vi "Test Deserialize Floating Point.vi"(8 "error in (no error)":errorcluster) -> (0 "error out":errorcluster)   [LabVIEW 2013]
uses:
  src/Deserializer/JSON Deserializer/JSON Deserializer.lvclass
  <vilib>/addons/_JKI Toolkits/Caraya/classes/Test/Test.lvclass
  <vilib>/addons/_JKI Toolkits/Caraya/classes/Assert/Assert.lvclass
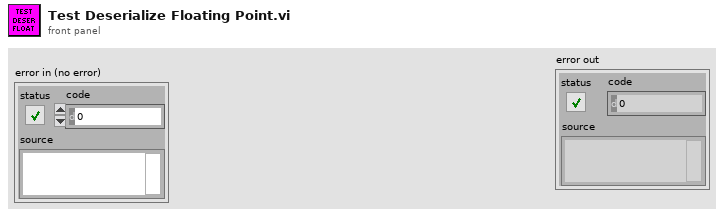
[diagram p1: front panel]
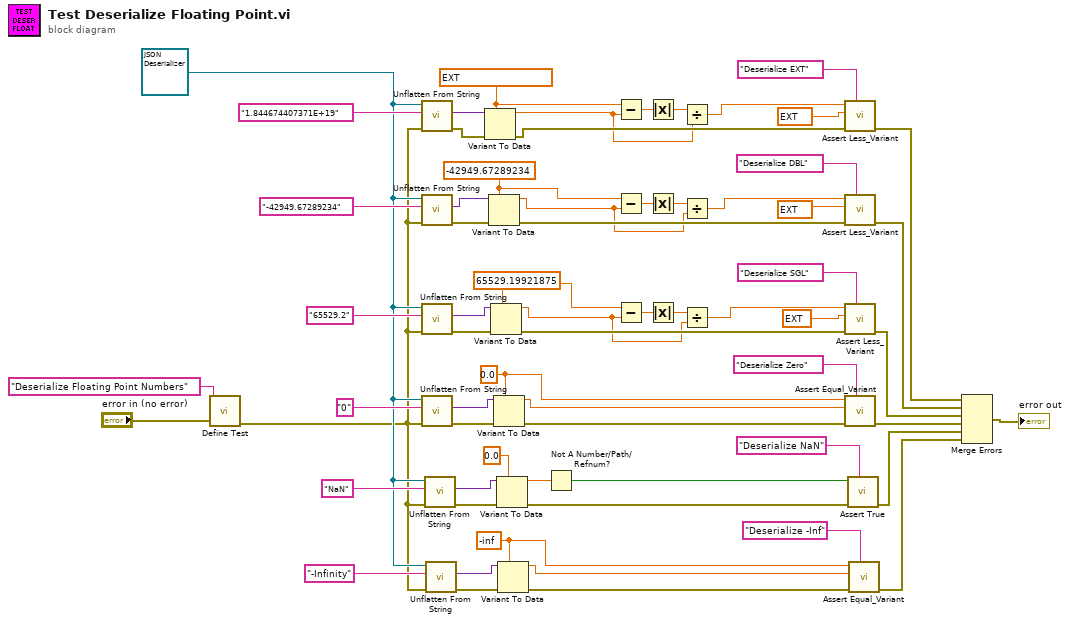
[diagram p0: block diagram]
diagram:
  w8 = -inf ("default (0 DBL)")
  w6 = refnum<class "JSON Deserializer.lvclass"> refnum ("JKI JSON Serialization.lvlib:JSON Deserializer.lvclass")
  w35 = ext 1.844674407371e+19 ("default (0 DBL)")
  w31 = -42949.67289234 ("default (0 DBL)")
  w25 = sgl 65529.2 ("default (0 DBL)")
  w22 = 0.0 ("default (0 DBL)")
  n1 = call <vilib>:"Define Test.vi"("error in (no error)"="error in (no error)", "Label (VI Title)"="Deserialize Floating Point Numbers") -> ("error out"=w5:errorcluster)  [unwired: 9 in]
  n2 = call-dynamic "Unflatten From String.vi"("error in (no error)"=w5, "String"="1.844674407371E+19", "Deserializer in"=w6) -> ("error out"=w37:errorcluster, "Variant"=w38:variant)  [unwired: 6 in, 1 out]
  n3 = call-dynamic "Unflatten From String.vi"("error in (no error)"=w5, "String"="-42949.67289234", "Deserializer in"=w6) -> ("error out"=w61:errorcluster, "Variant"=w32:variant)  [unwired: 6 in, 1 out]
  n4 = call-dynamic "Unflatten From String.vi"("error in (no error)"=w5, "String"="65529.2", "Deserializer in"=w6) -> ("error out"=w63:errorcluster, "Variant"=w27:variant)  [unwired: 6 in, 1 out]
  n5 = call-dynamic "Unflatten From String.vi"("error in (no error)"=w5, "String"="0", "Deserializer in"=w6) -> ("error out"=w65:errorcluster, "Variant"=w23:variant)  [unwired: 6 in, 1 out]
  n6 = call-dynamic "Unflatten From String.vi"("error in (no error)"=w5, "String"="NaN", "Deserializer in"=w6) -> ("error out"=w19:errorcluster, "Variant"=w16:variant)  [unwired: 6 in, 1 out]
  n7 = call-dynamic "Unflatten From String.vi"("error in (no error)"=w5, "String"="-Infinity", "Deserializer in"=w6) -> ("error out"=w11:errorcluster, "Variant"=w9:variant)  [unwired: 6 in, 1 out]
  n8 = Variant To Data(error in=w37, type=w35, Variant=w38) -> (data=w34:ext, error out=w36:errorcluster)
  n9 = Variant To Data(error in=w61, type=w31, Variant=w32) -> (data=w29:dbl, error out=w33:errorcluster)
  n10 = Variant To Data(error in=w63, type=w25, Variant=w27) -> (data=w26:sgl, error out=w28:errorcluster)
  n11 = Variant To Data(error in=w65, type=w22, Variant=w23) -> (data=w20:dbl, error out=w24:errorcluster)
  n12 = Variant To Data(error in=w19, type=0.0 ("default (0 DBL)"), Variant=w16) -> (data=w12:dbl, error out=w17:errorcluster)
  n13 = Variant To Data(error in=w11, type=w8, Variant=w9) -> (data=w2:dbl, error out=w10:errorcluster)
  n14 = Not A Number/Path/Refnum?(number/path/refnum=w12) -> (NaN/Path/Refnum?=w1:bool)
  n15 = Subtract(x=w35, y=w34) -> (x-y=w52:ext)
  n16 = Subtract(x=w31, y=w29) -> (x-y=w51:dbl)
  n17 = Subtract(x=w25, y=w26) -> (x-y=w50:sgl)
  n18 = Absolute Value(x=w52) -> (abs(x)=w49:ext)
  n19 = Absolute Value(x=w51) -> (abs(x)=w48:dbl)
  n20 = Absolute Value(x=w50) -> (abs(x)=w47:sgl)
  n21 = Divide(x=w49, y=w34) -> (x/y=w46:ext)
  n22 = Divide(x=w48, y=w29) -> (x/y=w45:dbl)
  n23 = Divide(x=w47, y=w26) -> (x/y=w44:sgl)
  n24 = call <vilib>:"Assert Less_Variant.vi"("Label"="Deserialize EXT", "error in (no error)"=w36, "Y"=ext 1e-13 ("default (0 DBL)"), "X"=w46) -> ("error out"=w54:errorcluster)  [unwired: 7 in]
  n25 = call <vilib>:"Assert Less_Variant.vi"("Label"="Deserialize DBL", "error in (no error)"=w33, "Y"=ext 1e-11 ("default (0 DBL)"), "X"=w45) -> ("error out"=w55:errorcluster)  [unwired: 7 in]
  n26 = call <vilib>:"Assert Less_Variant.vi"("Label"="Deserialize SGL", "error in (no error)"=w28, "Y"=ext 0.00001 ("default (0 DBL)"), "X"=w44) -> ("error out"=w56:errorcluster)  [unwired: 7 in]
  n27 = call <vilib>:"Assert Equal_Variant.vi"("Label"="Deserialize Zero", "error in (no error)"=w24, "Y"=w20, "X"=w22) -> ("error out"=w57:errorcluster)  [unwired: 7 in]
  n28 = call <vilib>:"Assert True.vi"("Label"="Deserialize NaN", "error in (no error)"=w17, "True?"=w1) -> ("error out"=w13:errorcluster)  [unwired: 8 in]
  n29 = call <vilib>:"Assert Equal_Variant.vi"("Label"="Deserialize -Inf", "error in (no error)"=w10, "Y"=w2, "X"=w8) -> ("error out"=w4:errorcluster)  [unwired: 7 in]
  n30 = Merge Errors(w54, w55, w56, w57, w13, w4) -> (→"error out":errorcluster)
